vi "lsl remove child n.vi"(8 "error in (no error)":errorcluster, 10 "name":string, 11 "e":cluster{}) -> (0 "error out":errorcluster, 3 "e out":cluster{})   [LabVIEW 2018, in "liblsl-LabVIEW.lvlib"]
doc: "extern LIBLSL_C_API void lsl_remove_child_n(lsl_xml_ptr e, const char *name);"
uses:
  <userlib>/liblsl-LabVIEW/liblsl-LabVIEW.lvlib
  <userlib>/liblsl-LabVIEW/liblsl64.dll
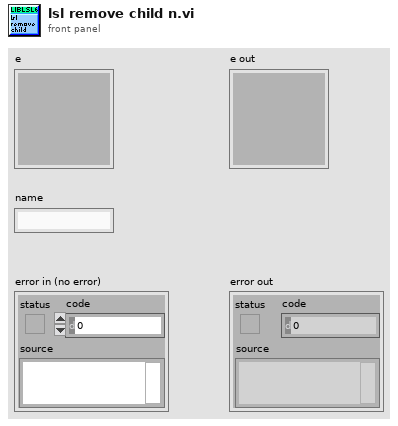
[diagram p1: front panel]
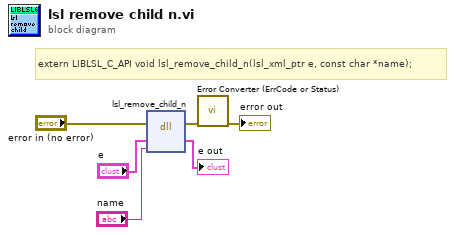
[diagram p0: block diagram]
diagram:
  # "extern LIBLSL_C_API void lsl_remove_child_n(lsl_xml_ptr e, const char *name);"
  n1 = dll-call lib="C:/Program Files/National Instruments/LabVIEW 2018/user.lib/liblsl-LabVIEW/liblsl64.*" fn="lsl_remove_child_n"(error in="error in (no error)", "e"="e", "name"="name") -> (error out=w2:errorcluster, "e"=→"e out":cluster{})  [unwired: 4 in, 1 out]
  n2 = call <userlib>:"Error Converter (ErrCode or Status).vi"("error in (no error)"=w2) -> ("error out"=→"error out":errorcluster)  [unwired: 10 in]
